vi "processString.vi"(8 "error in (no error)":errorcluster, 10 "Message in":string, 11 "Sent message in":refnum<class "VariantMessage.lvclass">) -> (0 "error out":errorcluster, 1 "found?":bool, 2 "response":T1, 3 "Sent message out":refnum<class "VariantMessage.lvclass">, 4 "isAck?":bool, 5 "Remaining buffer":string)   [LabVIEW 2025, in "VariantMessage.lvclass"]
doc: "Parses and interpretes the input string. If a complete packet from the remote host is found, \"found?\" should return TRUE. In that the case, the response should contain the type and the message data in the variant. \nIf the found message is an acknowledgement to the \"Sent message in\", the isAck? boolean should return TRUE.\nAnything left in the Message in string after the first message has been found should be returned in Remaining buffer"
uses:
  VariantMessage.lvclass
  response.ctl
  driver_status.ctl
  BaseMessage/BaseMessage.lvclass
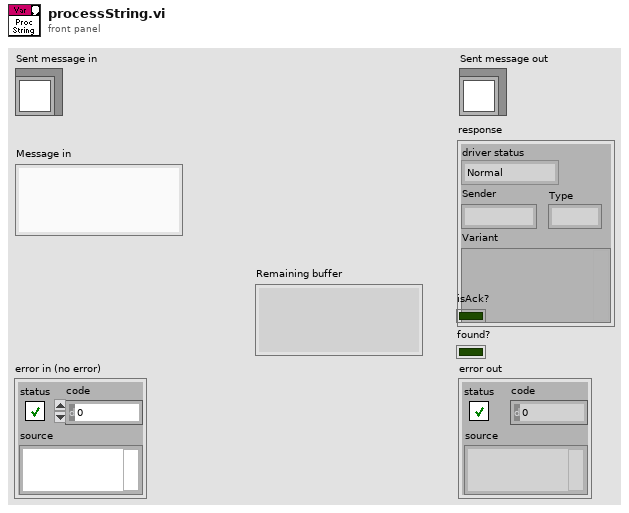
[diagram p1: front panel]
types:
  T1 = typedef "response.ctl" = cluster{"driver status":T2, "Sender":string, "Type":i32, "Variant":variant}
  T2 = typedef "driver_status.ctl" = enum16{"Normal", "Startup", "Connection lost", "Reconnected", "Timeout", "Idle", "Busy"}
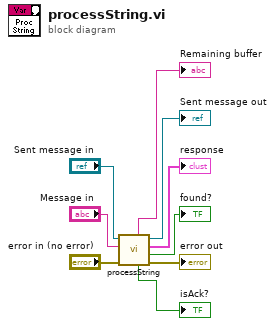
[diagram p0: block diagram]
diagram:
  n1 = call-parent "processString.vi"("error in (no error)"="error in (no error)", "Message in"="Message in", "Sent message in"="Sent message in") -> ("error out"=→"error out":errorcluster, "found?"=→"found?":bool, "response"=→"response":T1, "Sent message out"=→"Sent message out":refnum<class "VariantMessage.lvclass">, "isAck?"=→"isAck?":bool, "Remaining buffer"=→"Remaining buffer":string)  [unwired: 3 in]
